vi "SendBrakesCAN.vi"(8 "error in (no error)":errorcluster, 11 "interface object in":refnum<k20>) -> (0 "error out":errorcluster, 3 "interface object out":refnum<k20>)   [LabVIEW 2014]
uses:
  <vilib>/RioEmbeddedCAN/RioEmbeddedCAN.llb/CANFrameControl.ctl
  Global Data.vi
  <vilib>/RioEmbeddedCAN/RioEmbeddedCAN.llb/CANWaitTransmitComplete.vi
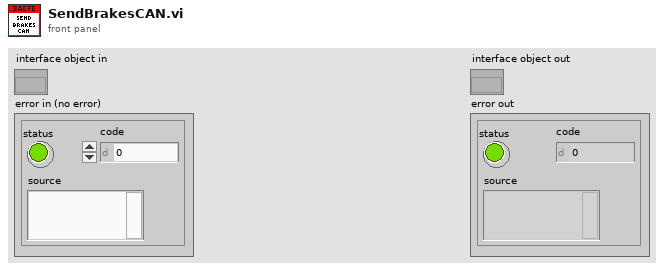
[diagram p1: front panel]
types:
  T1 = typedef "CANFrameControl.ctl" = cluster{"identifier":u32, "extended?":bool, "type":u8, "payload":u8[]}
  T2 = typedef "MC Temp 2.ctl" = cluster{"TMCControlBoard":dbl, "TMCRTD1":dbl, "TMCRTD2":dbl, "TMCRTD3":dbl}
  T3 = typedef "BMS Telemetry.ctl" = cluster{"bBMSIgnition":bool, "bBMSChargerMains":bool, "bBMSFastCharge":bool, "bBMSChargerEnabled":bool, "eBMSCarState":enum16{"Off", "On, Not Charging", "Charging", "Charging Finished", "Charging Error"}, "eBMSChargingState":enum16{"Disconnected", "Pre-charging", "Main Charging", "Balancing", "Charging Finished OK", "Charging Error"}, "tBMSChargeStage":u16, "eBMSLastChargeError":enum16{"No Error", "Cell Voltage Too Low", "No Comm from Cells so can't start", "Maximum charging stage duration expired", "No Comm from Cels so can't balande", "Cannot set balancing voltage", "Cell temps too high", "No Comms so can't determine temp", "# of Cells Mismatch", "Cells Overvoltage", "Cell Protection Event occured."}, "NBMSNumCells":u8, "bBMSUnderVProtection":bool, "bBMSOverVProtection":bool, "bBMSOverTProtection":bool, "bBMSLeakageProtection":bool, "bBMSNoCellCommsError":bool, "bBMSLowVReduction":bool, "bBMSHighTReduction":bool, "VCellMin":dbl, "VCellMax":dbl, "VCellMean":dbl, "VTotal":dbl, "TCellMin":dbl, "TCellMax":dbl, "TCellMean":dbl, "VCells":cluster{"[0]":dbl, "[1]":dbl, "[2]":dbl, "[3]":dbl, "[4]":dbl, "[5]":dbl, "[6]":dbl, "[7]":dbl, "[8]":dbl, "[9]":dbl, "[10]":dbl, "[11]":dbl, "[12]":dbl, "[13]":dbl, "[14]":dbl, "[15]":dbl, "[16]":dbl, "[17]":dbl, "[18]":dbl, "[19]":dbl, "[20]":dbl, "[21]":dbl, "[22]":dbl, "[23]":dbl, "[24]":dbl, "[25]":dbl, "[26]":dbl, "[27]":dbl, "[28]":dbl, "[29]":dbl, "[30]":dbl, "[31]":dbl, "[32]":dbl, "[33]":dbl, "[34]":dbl, "[35]":dbl, "[36]":dbl, "[37]":dbl, "[38]":dbl, "[39]":dbl, "[40]":dbl, "[41]":dbl, "[42]":dbl, "[43]":dbl, "[44]":dbl, "[45]":dbl, "[46]":dbl, "[47]":dbl, "[48]":dbl, "[49]":dbl, "[50]":dbl, "[51]":dbl, "[52]":dbl, "[53]":dbl, "[54]":dbl, "[55]":dbl, "[56]":dbl, "[57]":dbl, "[58]":dbl, "[59]":dbl, "[60]":dbl, "[61]":dbl, "[62]":dbl, "[63]":dbl, "[64]":dbl, "[65]":dbl, "[66]":dbl, "[67]":dbl, "[68]":dbl, "[69]":dbl, "[70]":dbl}, "TCells":cluster{"[0]":dbl, "[1]":dbl, "[2]":dbl, "[3]":dbl, "[4]":dbl, "[5]":dbl, "[6]":dbl, "[7]":dbl, "[8]":dbl, "[9]":dbl, "[10]":dbl, "[11]":dbl, "[12]":dbl, "[13]":dbl, "[14]":dbl, "[15]":dbl, "[16]":dbl, "[17]":dbl, "[18]":dbl, "[19]":dbl, "[20]":dbl, "[21]":dbl, "[22]":dbl, "[23]":dbl, "[24]":dbl, "[25]":dbl, "[26]":dbl, "[27]":dbl, "[28]":dbl, "[29]":dbl, "[30]":dbl, "[31]":dbl, "[32]":dbl, "[33]":dbl, "[34]":dbl, "[35]":dbl, "[36]":dbl, "[37]":dbl, "[38]":dbl, "[39]":dbl, "[40]":dbl, "[41]":dbl, "[42]":dbl, "[43]":dbl, "[44]":dbl, "[45]":dbl, "[46]":dbl, "[47]":dbl, "[48]":dbl, "[49]":dbl, "[50]":dbl, "[51]":dbl, "[52]":dbl, "[53]":dbl, "[54]":dbl, "[55]":dbl, "[56]":dbl, "[57]":dbl, "[58]":dbl, "[59]":dbl, "[60]":dbl, "[61]":dbl, "[62]":dbl, "[63]":dbl, "[64]":dbl, "[65]":dbl, "[66]":dbl, "[67]":dbl, "[68]":dbl, "[69]":dbl, "[70]":dbl}}
  T4 = typedef "MC Temp 1.ctl" = cluster{"TMCModuleA":dbl, "TMCModuleB":dbl, "TMCModuleC":dbl, "TMCGateDriver":dbl}
  T5 = typedef "MC Temp 3.ctl" = cluster{"TMCRTD4":dbl, "TMCRTD5":dbl, "TMotor":dbl, "MTorqueShudder":dbl}
  T6 = typedef "FPGA Telemetry.ctl" = cluster{"CPU Load":cluster{"Total (%)":dbl, "Time Critical (%)":dbl, "Timed Structures (%)":dbl, "High (%)":dbl, "Above Normal (%)":dbl, "Normal (%)":dbl, "Background (%)":dbl, "Idle (%)":dbl, "ISR (%)":dbl}, "SVehicleStatus":cluster{"BMS Status":T7, "MC Status":T7, "Shutdown Status":T7, "sbRIO Status":T7, "Vehicle Status":T7, "Shutdown State":T10, "AIR Status":T11, "Remote Return to Pits":bool, "Reason for Shutdown":T12, "MC State Machine Status":T13}, "iPhone HF Data":cluster{"gXiPhone":dbl, "gYiPhone":dbl, "gZiPhone":dbl, "nYawXiPhone":dbl, "nYawYiPhone":dbl, "nYawZiPhone":dbl}, "iPhone LF Data":cluster{"nLatiPhone":dbl, "nLongiPhone":dbl, "nGPSiPhone":dbl}, "stop":bool, "VSupplyOffset":fxp<+,12,4>, "VsbRIOSupply":fxp<+/-,25,6>, "bFPGALED":bool, "TSBRIO":fxp<+/-,33,17>, "rTPS2Unscaled":fxp<+/-,16,1>, "rTPS1Unscaled":fxp<+/-,16,1>, "bTPSConsistent":bool, "bTPSInRange":bool, "rThrottle":fxp<+/-,33,22>, "VTPS2":fxp<+/-,24,5>, "rTPS2":fxp<+/-,31,22>, "VTPS1":fxp<+/-,24,5>, "rTPS1":fxp<+/-,31,22>, "rTPS2Max":fxp<+,16,4>, "rTPS2Min":fxp<+,16,4>, "rTPS1Max":fxp<+,16,4>, "rTPS1Min":fxp<+,16,4>, "bCoolantPumpEnable":bool, "bRTDSEnable":bool, "bTSMSInStatus":bool, "bPosAIREnable":bool, "bBMSOK":bool, "bIMDOK":bool, "bBSPDOK":bool, "bSBRIOOK2":bool, "bSBRIOOK1":bool, "bTSMSOutStatus":bool, "eGreenDash":T14, "eYellowDash":T14, "eRedDash":T14, "bMotorControllerEnable":bool, "tCurrentLap":u32, "bNewLap":bool, "tLastLap":u32, "tLapMin":u32, "V5VSupply":fxp<+/-,24,5>, "bWheelRL":bool, "bWheelRR":bool, "bWheelFR":bool, "bWheelFL":bool, "VBrakePressureR":fxp<+/-,24,5>, "VBrakePressureF":fxp<+/-,24,5>, "bWheelRRStopped":bool, "bWheelRLStopped":bool, "bWheelFRStopped":bool, "bWheelFLStopped":bool, "tWheelRLPeriod":u32, "tWheelRRPeriod":u32, "tWheelFRPeriod":u32, "tWheelFLPeriod":u32, "bBrakeLight":bool, "VShockRR":fxp<+/-,24,5>, "VShockRL":fxp<+/-,24,5>, "VShockFR":fxp<+/-,24,5>, "VShockFL":fxp<+/-,24,5>, "IHighCurrent":fxp<+/-,24,15>, "ILowCurrent":fxp<+/-,24,15>, "pBrakeR":fxp<+,26,13>, "pBrakeF":fxp<+,26,13>, "bHighCurrentOK":bool, "bLowCurrentOK":bool, "bBrakeROK":bool, "bBrakeFOK":bool, "VSteerWheelMiddle":fxp<+/-,26,5>, "aSteerWheel":fxp<+/-,31,13>, "nWheelFL":fxp<+/-,32,16>, "nWheelFR":fxp<+/-,32,16>, "nWheelRL":fxp<+/-,32,16>, "nWheelRR":fxp<+/-,32,16>, "ADXL345 Output":T15, "Tire Diameter(m)":fxp<+,16,1>, "vWheelRR":fxp<+/-,32,18>, "vWheelRL":fxp<+/-,32,18>, "vWheelFR":fxp<+/-,32,18>, "vWheelFL":fxp<+/-,32,18>, "vWheelLowest":fxp<+/-,32,18>, "vWheelHighest":fxp<+/-,32,18>, "bAccel":bool, "vAxleF":fxp<+/-,33,19>, "vCar":fxp<+/-,33,19>, "sLap":fxp<+,32,12>, "rSlipRL":fxp<+/-,12,1>, "rSlipRR":fxp<+/-,12,1>, "rSlipFL":fxp<+/-,12,1>, "rSlipFR":fxp<+/-,12,1>, "NLap":u8, "tLapReference":u32, "tFastestLap":u32}
  T7 = typedef "Subsystem Status.ctl" = cluster{"eStatusSeverity":T8, "NValue":sgl, "CMessage":T9, "bNotOK":bool}
  T8 = typedef "Subsystem Status Severity.ctl" = enum16{"Okay", "Short Warning", "Long Warning", "Return to Pits", "Error", "Danger"}
  T9 = typedef "Subsystem Status Message.ctl" = enum16{"ControllerTemperature", "MotorTemperature", "BatteryTemperature", "BatteryLowVoltage", "LVBattery", "sbRIOTemperature", "Precharge", "BSPD", "IMD", "RemoteReturnToPits", "EStopInterrupted", "NoCellComms", "MCOverSpeed", "MCOverCurrent", "MCOverVoltage", "MCInverterOverTemp", "MCDirectionCommand", "MCInverterTimeout", "MCDesatFault", "MCHWOverCurrent", "MCUnderVoltage", "MCCommandMessageLost", "MotorOverTemp", "MCModAOverTemp", "MCModBOverTemp", "MCModCOverTemp", "MCPCBOverTemp", "MCGateDrv1OverTemp", "MCDateDrv2OverTemp", "MCCurrentSensorFault", "MCResolverNotConnected", "ShutdownLatchTripped", "UnknownBMS", "RemoteEmergency"}
  T10 = typedef "Shutdown State Machine.lvsc/State.ctl" = enum16{"NI.SC.Initial", "NI.SC.History", "NI.SC.ShallowHistory", "NI.SC.Terminal", "Coolant Pump Started/AIR's On", "AIRs On", "Precharge", "TSMS Off"}
  T11 = typedef "AIR Status.ctl" = enum16{"Off", "Precharge", "On"}
  T12 = typedef "Reason for Shutdown.ctl" = enum16{"None", "BMS", "Shutdown", "sbRIO", "MC", "Remote"}
  T13 = typedef "MC State Machine.lvsc/State.ctl" = enum16{"NI.SC.Initial", "NI.SC.History", "NI.SC.ShallowHistory", "NI.SC.Terminal", "Let Current Drop then Disable AIR's", "Enabled", "Disabled"}
  T14 = typedef "Dash LED Status.ctl" = enum16{"Off", "Flashing", "On"}
  T15 = typedef "ADXL345 Output.ctl" = cluster{"X":fxp<+/-,14,4>, "Y":fxp<+/-,14,4>, "Z":fxp<+/-,14,4>}
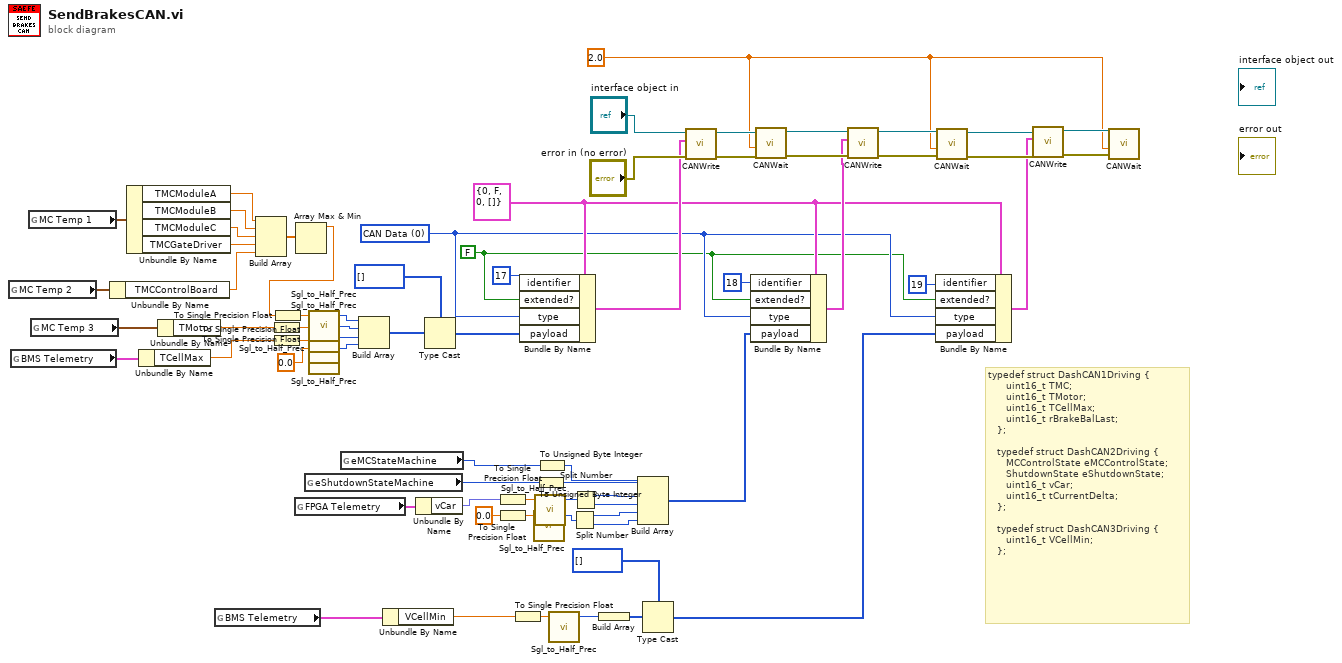
[diagram p0: block diagram]
diagram:
  w55 = 2.0
  w49 = u8 0 items=["CAN Data", "CAN Remote"] ("type")
  w53 = T1 {"identifier"=0, "extended?"=FALSE, "type"=0, "payload"=[]} ("CAN frame")
  w48 = FALSE ("extended?")
  # "typedef struct DashCAN1Driving {\n      uint16_t TMC;\n      uint16_t TMotor;\n      uint16_t TCellMax;\n      uint16_t rBrakeBalLast;\n   };\n\n   typedef struct DashCAN2Driving {\n      MCControlState eMCControlState;\n      ShutdownState eShutdownState;\n      uint16_t vCar;\n      uint16_t tCurrentDelta;\n   };\n\n   typedef struct DashCAN3Driving {\n      uint16_t VCellMin;\n   };"
  n1 = global read "Global Data.vi" "MC Temp 2"() -> (w36:T2)
  n2 = global read "Global Data.vi" "BMS Telemetry"() -> (w27:T3)
  n3 = global read "Global Data.vi" "MC Temp 1"() -> (w37:T4)
  n4 = global read "Global Data.vi" "MC Temp 3"() -> (w40:T5)
  n5 = Unbundle By Name(w36) -> ("TMCControlBoard"=w31:dbl)
  n6 = Unbundle By Name(w37) -> ("TMCModuleA"=w35:dbl, "TMCModuleB"=w34:dbl, "TMCModuleC"=w33:dbl, "TMCGateDriver"=w32:dbl)
  n7 = Unbundle By Name(w27) -> ("TCellMax"=w25:dbl)
  n8 = Unbundle By Name(w40) -> ("TMotor"=w39:dbl)
  n9 = global read "Global Data.vi" "BMS Telemetry"() -> (w16:T3)
  n10 = Build Array(w35, w34, w33, w32, w31) -> (w30:dbl[])
  n11 = To Single Precision Float(number=w39) -> (single precision float=w38:sgl)
  n12 = To Single Precision Float(number=w25) -> (single precision float=w26:sgl)
  n13 = global read "Global Data.vi" "FPGA Telemetry"() -> (w3:T6)
  n14 = Array Max & Min(array=w30) -> (max value=w28:dbl)  [unwired: 3 out]
  n15 = To Single Precision Float(number=w28) -> (single precision float=w29:sgl)
  n16 = global read "Global Data.vi" "eShutdownStateMachine"() -> (w4:T10)
  n17 = call "Sgl_to_Half_Prec.vi"("SGL"=w29) -> ("Half Precision Floating Point"=w44:u16)  [unwired: 4 in]
  n18 = call "Sgl_to_Half_Prec.vi"("SGL"=w38) -> ("Half Precision Floating Point"=w43:u16)  [unwired: 4 in]
  n19 = call "Sgl_to_Half_Prec.vi"("SGL"=w26) -> ("Half Precision Floating Point"=w42:u16)  [unwired: 4 in]
  n20 = call "Sgl_to_Half_Prec.vi"("SGL"=sgl 0.0) -> ("Half Precision Floating Point"=w41:u16)  [unwired: 4 in]
  n21 = global read "Global Data.vi" "eMCStateMachine"() -> (w5:T13)
  n22 = Build Array(w44, w43, w42, w41) -> (w45:u16[])
  n23 = Unbundle By Name(w16) -> ("VCellMin"=w15:dbl)
  n24 = Unbundle By Name(w3) -> ("vCar"=w2:fxp<+/-,33,19>)
  n25 = Type Cast(type=u8[] [], x=w45) -> (*(type *) &x=w47:u8[])
  n26 = To Single Precision Float(number=w2) -> (single precision float=w23:sgl)
  n27 = To Single Precision Float(number=sgl 0.0) -> (single precision float=w22:sgl)
  n28 = To Single Precision Float(number=w15) -> (single precision float=w19:sgl)
  n29 = Bundle By Name(cluster=w53, "identifier"=u32 17, "extended?"=w48, "type"=w49, "payload"=w47) -> (w66:T1)
  n30 = call "Sgl_to_Half_Prec.vi"("SGL"=w22) -> ("Half Precision Floating Point"=w14:u16)  [unwired: 4 in]
  n31 = call "Sgl_to_Half_Prec.vi"("SGL"=w23) -> ("Half Precision Floating Point"=w13:u16)  [unwired: 4 in]
  n32 = To Unsigned Byte Integer(number=w4) -> (unsigned 8bit integer=w11:u8)
  n33 = To Unsigned Byte Integer(number=w5) -> (unsigned 8bit integer=w12:u8)
  n34 = call "Sgl_to_Half_Prec.vi"("SGL"=w19) -> ("Half Precision Floating Point"=w20:u16)  [unwired: 4 in]
  n35 = Split Number(x=w14) -> (hi(x)=w8:u8, lo(x)=w7:u8)
  n36 = Split Number(x=w13) -> (hi(x)=w10:u8, lo(x)=w9:u8)
  n37 = Build Array(w20) -> (w21:u16[])
  n38 = Build Array(w12, w11, w10, w9, w8, w7) -> (w6:u8[])
  n39 = Type Cast(type=u8[] [], x=w21) -> (*(type *) &x=w17:u8[])
  n40 = call <vilib>:"CANWrite.vi"("error in (no error)"="error in (no error)", "CAN frame"=w66, "interface object in"="interface object in") -> ("error out"=w64:errorcluster, "interface object out"=w65:refnum<k20>)  [unwired: 7 in]
  n41 = Bundle By Name(cluster=w53, "identifier"=u32 18, "extended?"=w48, "type"=w49, "payload"=w6) -> (w54:T1)
  n42 = call-poly <vilib>:"CANWait.vi"("error in (no error)"=w64, "timeout (0 s)"=w55, "interface object in"=w65) -> ("error out"=w62:errorcluster, "interface object out"=w63:refnum<k20>)  [unwired: 7 in]
  n43 = call <vilib>:"CANWrite.vi"("error in (no error)"=w62, "CAN frame"=w54, "interface object in"=w63) -> ("error out"=w60:errorcluster, "interface object out"=w61:refnum<k20>)  [unwired: 7 in]
  n44 = Bundle By Name(cluster=w53, "identifier"=u32 19, "extended?"=w48, "type"=w49, "payload"=w17) -> (w52:T1)
  n45 = call-poly <vilib>:"CANWait.vi"("error in (no error)"=w60, "timeout (0 s)"=w55, "interface object in"=w61) -> ("error out"=w58:errorcluster, "interface object out"=w59:refnum<k20>)  [unwired: 7 in]
  n46 = call <vilib>:"CANWrite.vi"("error in (no error)"=w58, "CAN frame"=w52, "interface object in"=w59) -> ("error out"=w56:errorcluster, "interface object out"=w57:refnum<k20>)  [unwired: 7 in]
  n47 = call-poly <vilib>:"CANWait.vi"("error in (no error)"=w56, "timeout (0 s)"=w55, "interface object in"=w57) -> ()  [unwired: 7 in, 2 out]
